vi "BasicWrite.vi"() -> ()   [LabVIEW 2015, in "AODControl.lvlib"]
uses:
  AODControl.lvlib
panel:
  in  "stop":bool
  out "Array":u32[](array[numeric]) format="%x"
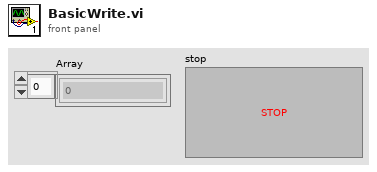
[diagram p1: front panel]
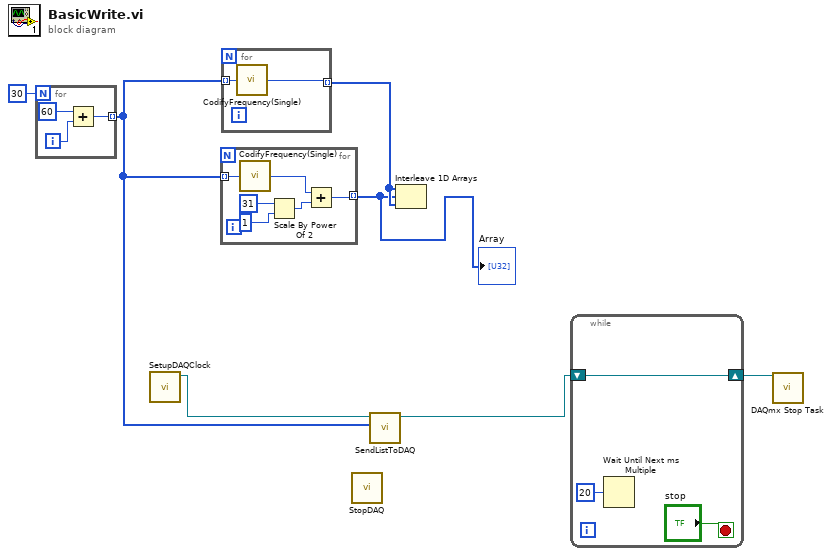
[diagram p0: block diagram]
diagram:
  n1 = for {
    N: 30 -> [_]
    tunnel: [w8] -> w3 mode=indexing
    i -> [w10]
    n2 = Add(x=60, y=w10) -> (x+y=w8:i32)
  }
  n3 = call "SetupDAQClock.vi"() -> ("task out"=w1:refnum<k21>)  [unwired: 10 in, 1 out]
  n4 = for {
    tunnel: w3 -> [w12] mode=indexing
    tunnel: [w11] -> w2 mode=indexing
    n5 = call "CodifyFrequency(Single).vi"("Frequency In"=w12) -> ("32bit integer"=w16:u32)
    n6 = Scale By Power Of 2(n=i16 31, x=u32 1 ("32bit integer")) -> (x*2^n=w13:u32)
    n7 = Add(x=w16, y=w13) -> (x+y=w11:u32)
  }
  "Array" <- w2
  n8 = for {
    tunnel: w3 -> [w18] mode=indexing
    tunnel: [w17] -> w5 mode=indexing
    n9 = call "CodifyFrequency(Single).vi"("Frequency In"=w18) -> ("32bit integer"=w17:u32)
  }
  n10 = call "StopDAQ.vi"() -> ()  [unwired: 11 in, 1 out]
  n11 = call "SendListToDAQ.vi"("Input"=w3, "Refnum in"=w1) -> ("Refnum out"=w4:refnum<k21>)  [unwired: 8 in, 1 out]
  n12 = Interleave 1D Arrays(w5, w2, w5) -> ()  [unwired: 1 out]
  n13 = while {
    shift-right: [w19] -> w7
    shift-left: w4 -> [w19]
    stop <- "stop" stop-if-true
    n14 = Wait Until Next ms Multiple(millisecond multiple=u32 20) -> ()  [unwired: 1 out]
  }
  n15 = call <vilib>:"DAQmx Stop Task.vi"("task/channels in"=w7) -> ()  [unwired: 13 in, 2 out]
